vi "Write ITX (R+coord).vi"(10 "coordinates file path":path, 11 "ibw file path":path=path "C:/Work/IBW - LVArray/BTOCu1005.ibw") -> ()   [LabVIEW 2020, in "Data.ITX.lvclass"]
uses:
  Data.ITX.lvclass
  <vilib>/Utility/file.llb/Read Delimited Spreadsheet (string).vi
  <vilib>/Utility/file.llb/Read Delimited Spreadsheet (DBL).vi
  Data/Data.lvclass
panel:
  in  "Commands":string
  in  "Notes":string
  out "String":string
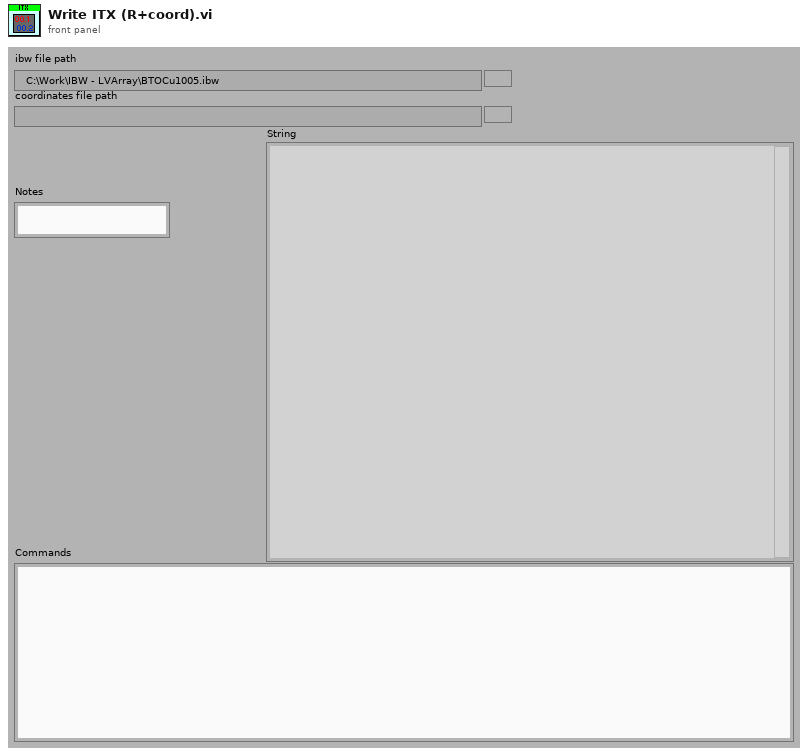
[diagram p1: front panel]
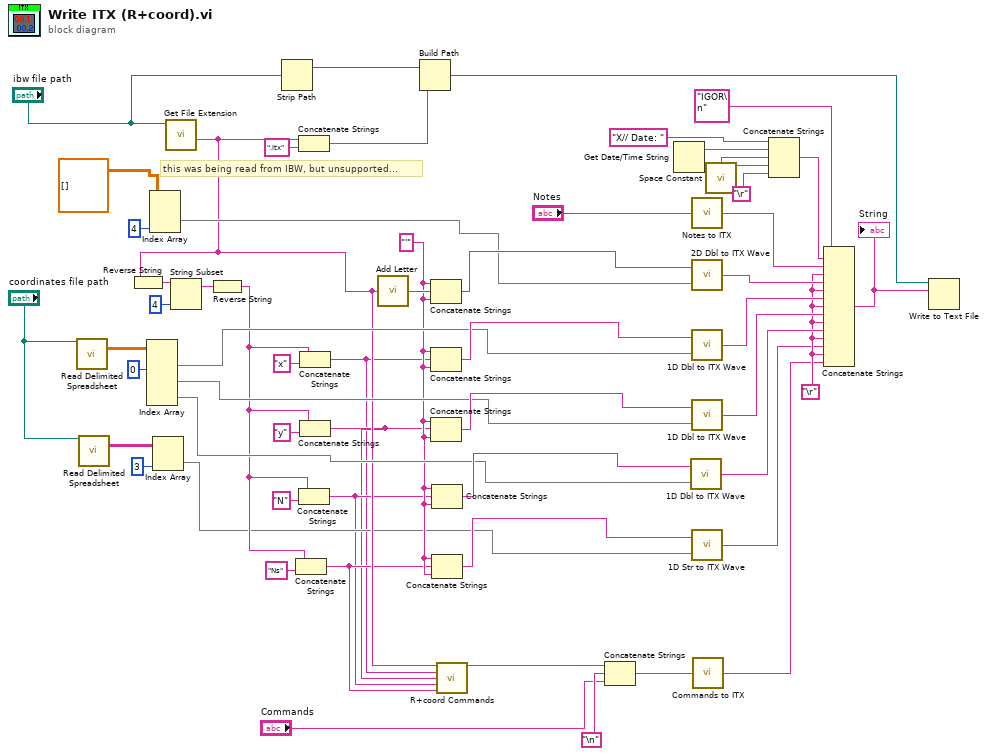
[diagram p0: block diagram]
diagram:
  w19 = "'" ("string")
  w23 = "\r"
  # "this was being read from IBW, but unsupported..."
  n1 = call-poly <vilib>:"Read Delimited Spreadsheet.vi"("file path (dialog if empty)"="coordinates file path") -> ("all rows"=w34:dbl[][])  [unwired: 9 in, 5 out]
  n2 = call-poly <vilib>:"Read Delimited Spreadsheet.vi"("file path (dialog if empty)"="coordinates file path") -> ("all rows"=w2:string[][])  [unwired: 9 in, 5 out]
  n3 = Index Array(array=w34, index (col) #1=0 ("disabled index (col)")) -> (element #1=w30:dbl[], element #2=w31:dbl[], element #3=w32:dbl[])  [unwired: 5 in]
  n4 = Index Array(array=dbl[][][] [] ("Output Array"), index (dim 2)=4 ("disabled index (col)")) -> (element=w35:dbl[][])  [unwired: 2 in]
  n5 = Index Array(array=w2, index (col)=3 ("disabled index (col)")) -> (element=w7:string[])  [unwired: 1 in]
  n6 = call <vilib>:"Get File Extension.vi"("file"="ibw file path") -> ("filename without extension"=w13:string)  [unwired: 1 in, 9 out]
  n7 = Reverse String(1:w13) -> (0:w12:string)
  n8 = String Subset(string=w12, length (rest)=4 ("length (rest)")) -> (substring=w11:string)  [unwired: 1 out]
  n9 = Reverse String(1:w11) -> (0:w10:string)
  n10 = Strip Path(path="ibw file path") -> (stripped path=w16:path)  [unwired: 1 out]
  n11 = Concatenate Strings(w10, "Ns" ("string")) -> (w6:string)
  n12 = Concatenate Strings(w13, ".itx" ("string")) -> (w15:string)
  n13 = Concatenate Strings(w10, "N" ("string")) -> (w5:string)
  n14 = Concatenate Strings(w10, "x" ("string")) -> (w3:string)
  n15 = Concatenate Strings(w10, "y" ("string")) -> (w4:string)
  n16 = call "Add Letter.vi"("string"=w13) -> ("result string"=w42:string)
  n17 = Build Path(base path=w16, name or relative path=w15) -> (appended path=w14:path)
  n18 = Concatenate Strings(w19, w42, w19) -> (w39:string)
  n19 = Concatenate Strings(w19, w3, w19) -> (w40:string)
  n20 = Concatenate Strings(w19, w4, w19) -> (w41:string)
  n21 = Concatenate Strings(w19, w5, w19) -> (w37:string)
  n22 = Concatenate Strings(w19, w6, w19) -> (w20:string)
  n23 = call "R+coord Commands.vi"("2D wavename"=w13, "X wavename"=w3, "Y wavename"=w4, "N wavename"=w5, "Ns wavename"=w6) -> ("result string"=w38:string)  [unwired: 1 in, 9 out]
  n24 = Concatenate Strings(w38, "\n", "Commands") -> (w45:string)
  n25 = Get Date/Time String() -> (date string=w57:string, time string=w58:string)  [unwired: 3 out]
  n26 = call "1D Dbl to ITX Wave.vi"("1D Array"=w32, "Wavename"=w37) -> ("ITX Wave"=w24:string)
  n27 = call "Notes to ITX.vi"("Notes"="Notes") -> ("ITX Notes"=w49:string)
  n28 = call "2D Dbl to ITX Wave.vi"("2D Array"=w35, "Wavename"=w39) -> ("ITX Wave"=w52:string)
  n29 = call "1D Dbl to ITX Wave.vi"("1D Array"=w30, "Wavename"=w40) -> ("ITX Wave"=w51:string)
  n30 = call "1D Dbl to ITX Wave.vi"("1D Array"=w31, "Wavename"=w41) -> ("ITX Wave"=w50:string)
  n31 = call "1D Str to ITX Wave.vi"("String"=w7, "Wavename"=w20) -> ("ITX Wave"=w21:string)
  n32 = call "Commands to ITX.vi"("Commands"=w45) -> ("ITX Commands"=w22:string)
  n33 = call <vilib>:"Space Constant.vi"() -> ("String"=w47:string)
  n34 = Concatenate Strings("X// Date: " ("format string"), w57, w47, w58, "\r") -> (w56:string)
  n35 = Concatenate Strings("IGOR\n", w56, w49, w23, w52, w23, w51, w23, w50, w23, w24, w23, w21, w23, w22) -> (w48:string)
  "String" <- w48
  n36 = Write to Text File(file (use dialog)=w14, text=w48) -> ()  [unwired: 1 in, 4 out]
